vi "梦幻城堡C1~3界面.vi"() -> ()   [LabVIEW 2016, in "环境动力监测库.lvlib" / "UPS库.lvlib"]
uses:
  <vilib>/Utility/config.llb/NI_LVConfig.lvlib
  <vilib>/ptbypt/NI_PtbyPt.lvlib
panel:
  out "关机倒计时":i32
  out "关闭中":bool
  out "通信指示":bool
  out "UPS状态":T1
  in  "关机":bool
  in  "重开串口":bool
  out "Temperature":dbl
  out "Battery voltage":dbl
  out "I/P frequency HZ":dbl
  out "O/P load %":dbl
  out "O/P voltage":dbl
  out "I/P fault voltage":dbl
  out "I/P voltage":dbl
  # "UPS-梦幻城堡C1~3"
  # "输入电压V"
  # "输入故障电压V"
  # "输出电压V"
  # "输出电流A"
  # "输入频率HZ"
  # "电池电压V"
  # "UPS温度℃"
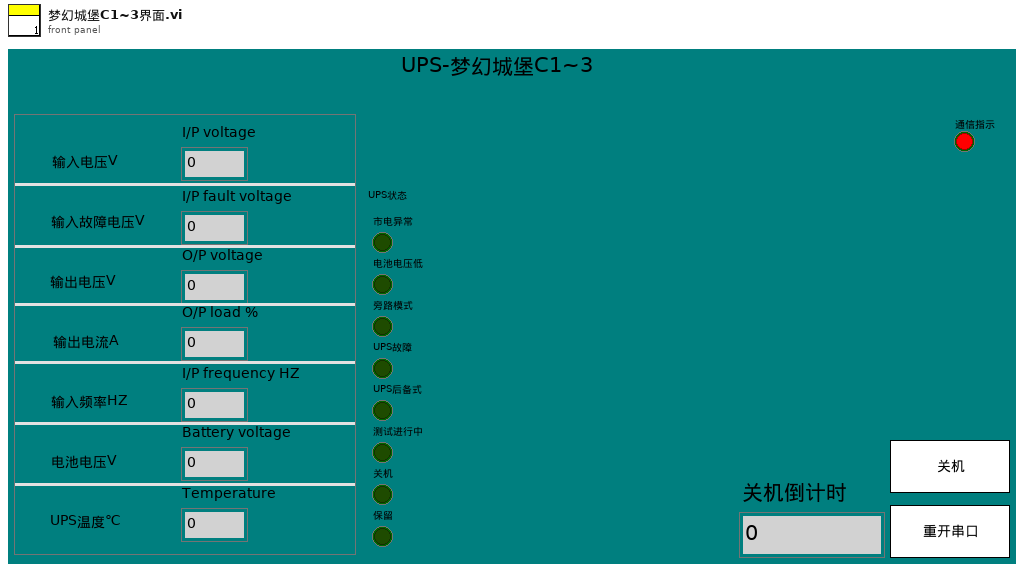
[diagram p1: front panel]
types:
  T1 = cluster{"市电异常":bool, "电池电压低":bool, "旁路模式":bool, "UPS故障":bool, "UPS后备式":bool, "测试进行中":bool, "关机":bool, "保留":bool}
  T2 = cluster{"枚举":enum16{"open", "read", "write", "close"}, "写入缓冲区":string}
  T3 = cluster{"时间标识":timestamp, "设备":string, "日志信息":string}
  T4 = cluster{"I/P voltage":dbl, "I/P fault voltage":dbl, "O/P voltage":dbl, "O/P load %":dbl, "I/P frequency HZ":dbl, "Battery voltage":dbl, "Temperature":dbl, "U":string}
  T5 = cluster{"[0]":bool, "[1]":bool, "[2]":bool, "[3]":bool, "[4]":bool, "[5]":bool, "[6]":bool, "[7]":bool}
  T6 = typedef "NI_LVConfig.lvlib/Config Data RefNum.ctl" = refnum<k1>
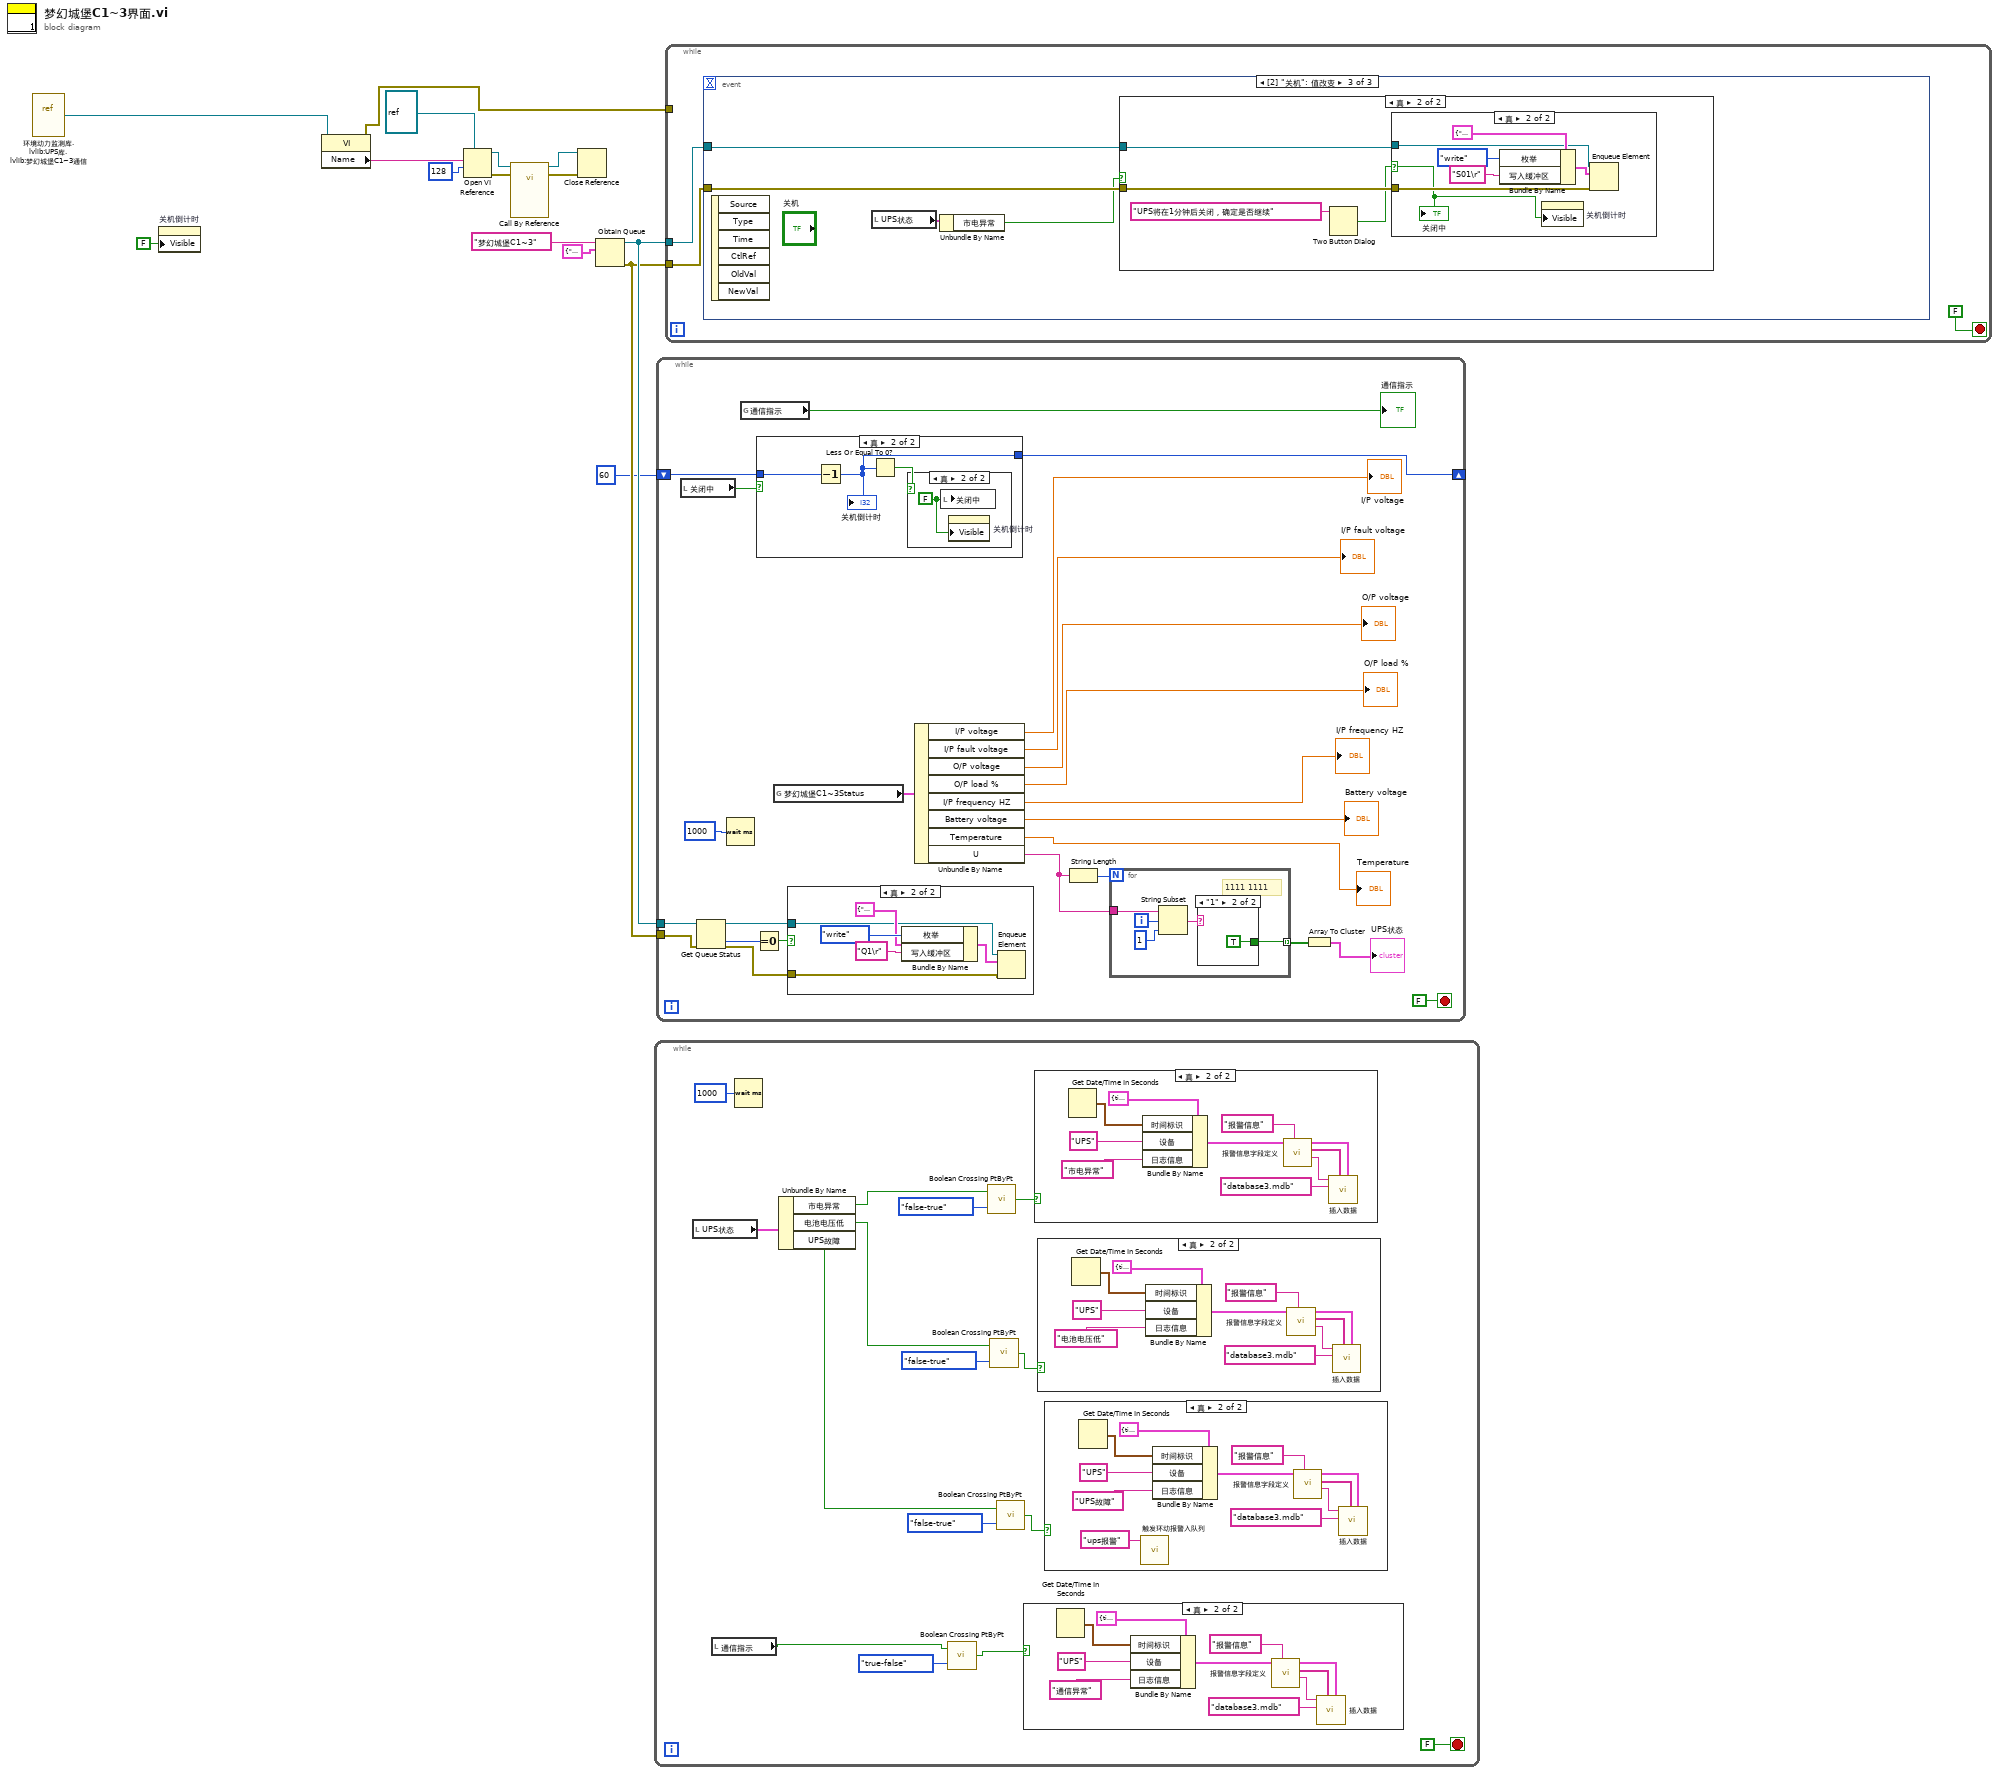
[diagram p0: block diagram]
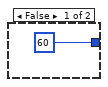
[diagram p7: hidden frame]
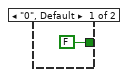
[diagram p9: hidden frame]
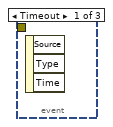
[diagram p10: hidden frame]
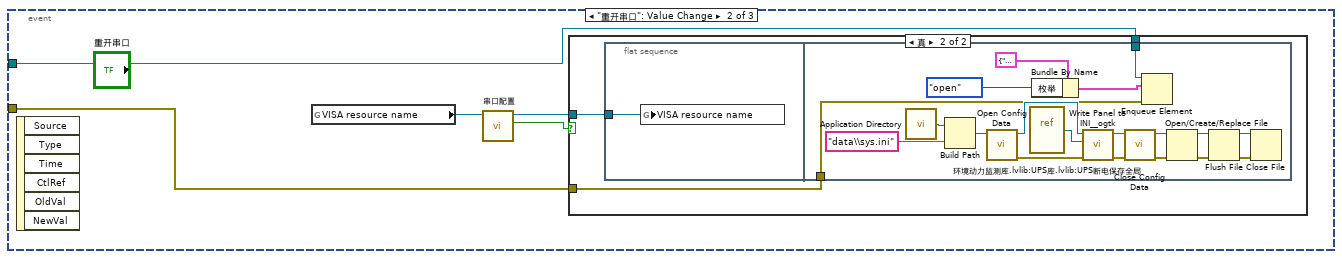
[diagram p11: hidden frame]
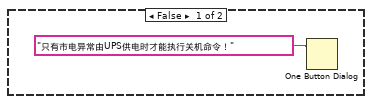
[diagram p13: hidden frame]
diagram:
  n1 = vi-ref "环境动力监测库.lvlib:UPS库.lvlib:梦幻城堡C1~3通信.vi"() -> (w8:refnum<vi>)
  n2 = property on="关机倒计时" class="DigNum (严格)"("Visible"=FALSE ("可见")) -> ()  [unwired: 2 in, 2 out]
  n3 = property class="VI"(reference=w8) -> (error out=w2:errorcluster, "Name"=w9:string)  [unwired: 1 in, 1 out]
  n4 = Open VI Reference(type specifier VI Refnum (for type only)=refnum<vi> refnum, vi path=w9, options=128 ("选项")) -> (vi reference=w11:refnum<vi>, error out=w13:errorcluster)  [unwired: 3 in]
  n5 = call-by-ref "?"(reference=w11, error in=w13) -> (reference out=w15:refnum<vi>, error out=w14:errorcluster)  [unwired: 12 in]
  n6 = Close Reference(reference=w15, error in (no error)=w14) -> ()  [unwired: 1 out]
  n7 = Obtain Queue(name (unnamed)="梦幻城堡C1~3" ("名称（未命名）"), element data type=T2 {"枚举"=enum."open", "写入缓冲区"=""}) -> (queue out=w5:refnum<queue>, error out=w4:errorcluster)  [unwired: 3 in, 1 out]
  n8 = while {
    stop <- FALSE stop-if-true
    n9 = local read "UPS状态"() -> (w28:T1)
    n10 = local read "通信指示"() -> (w16:bool)
    n11 = Wait (ms)(milliseconds to wait=u32 1000 ("等待时间（毫秒）")) -> ()  [unwired: 1 out]
    n12 = Unbundle By Name(w28) -> ("市电异常"=w25:bool, "电池电压低"=w20:bool, "UPS故障"=w19:bool)
    n13 = call <vilib>:"Boolean Crossing PtByPt.vi"("direction"=enum16{"either", "false-true", "true-false"}."true-false", "input"=w16) -> ("crossing"=w17:bool)  [unwired: 1 in]
    n14 = call <vilib>:"Boolean Crossing PtByPt.vi"("direction"=enum16{"either", "false-true", "true-false"}."false-true", "input"=w25) -> ("crossing"=w26:bool)  [unwired: 1 in]
    n15 = call <vilib>:"Boolean Crossing PtByPt.vi"("direction"=enum16{"either", "false-true", "true-false"}."false-true", "input"=w20) -> ("crossing"=w23:bool)  [unwired: 1 in]
    n16 = call <vilib>:"Boolean Crossing PtByPt.vi"("direction"=enum16{"either", "false-true", "true-false"}."false-true", "input"=w19) -> ("crossing"=w22:bool)  [unwired: 1 in]
    n17 = case shown="真" w17 {
      frame False {
      }
      frame True {
        n18 = Get Date/Time In Seconds() -> (seconds since 1Jan1904=w39:timestamp)
        n19 = Bundle By Name(cluster=T3 {"时间标识"=timestamp(0 s since 1904-01-01), "设备"="", "日志信息"=""} ("data in"), "时间标识"=w39, "设备"="UPS", "日志信息"="通信异常") -> (w38:T3)
        n20 = call "报警信息字段定义.vi"("table输入"="报警信息", "data in"=w38) -> ("table输出"=w34:string, "columns"=w33:string[], "data out"=w32:T3)  [unwired: 7 in]
        n21 = call "插入数据.vi"("data"=w32, "columns"=w33, "database"="database3.mdb", "table"=w34) -> ()  [unwired: 7 in, 1 out]
      }
    }
    n22 = case shown="真" w26 {
      frame False {
      }
      frame True {
        n23 = Get Date/Time In Seconds() -> (seconds since 1Jan1904=w70:timestamp)
        n24 = Bundle By Name(cluster=T3 {"时间标识"=timestamp(0 s since 1904-01-01), "设备"="", "日志信息"=""} ("data in"), "时间标识"=w70, "设备"="UPS", "日志信息"="市电异常") -> (w69:T3)
        n25 = call "报警信息字段定义.vi"("table输入"="报警信息", "data in"=w69) -> ("table输出"=w65:string, "columns"=w64:string[], "data out"=w63:T3)  [unwired: 7 in]
        n26 = call "插入数据.vi"("data"=w63, "columns"=w64, "database"="database3.mdb", "table"=w65) -> ()  [unwired: 7 in, 1 out]
      }
    }
    n27 = case shown="真" w23 {
      frame False {
      }
      frame True {
        n28 = Get Date/Time In Seconds() -> (seconds since 1Jan1904=w60:timestamp)
        n29 = Bundle By Name(cluster=T3 {"时间标识"=timestamp(0 s since 1904-01-01), "设备"="", "日志信息"=""} ("data in"), "时间标识"=w60, "设备"="UPS", "日志信息"="电池电压低") -> (w59:T3)
        n30 = call "报警信息字段定义.vi"("table输入"="报警信息", "data in"=w59) -> ("table输出"=w55:string, "columns"=w54:string[], "data out"=w53:T3)  [unwired: 7 in]
        n31 = call "插入数据.vi"("data"=w53, "columns"=w54, "database"="database3.mdb", "table"=w55) -> ()  [unwired: 7 in, 1 out]
      }
    }
    n32 = case shown="真" w22 {
      frame False {
      }
      frame True {
        n33 = Get Date/Time In Seconds() -> (seconds since 1Jan1904=w50:timestamp)
        n34 = call "触发环动报警入队列.vi"("报警内容"="ups报警") -> ()  [unwired: 11 in]
        n35 = Bundle By Name(cluster=T3 {"时间标识"=timestamp(0 s since 1904-01-01), "设备"="", "日志信息"=""} ("data in"), "时间标识"=w50, "设备"="UPS", "日志信息"="UPS故障") -> (w49:T3)
        n36 = call "报警信息字段定义.vi"("table输入"="报警信息", "data in"=w49) -> ("table输出"=w45:string, "columns"=w44:string[], "data out"=w43:T3)  [unwired: 7 in]
        n37 = call "插入数据.vi"("data"=w43, "columns"=w44, "database"="database3.mdb", "table"=w45) -> ()  [unwired: 7 in, 1 out]
      }
    }
  }
  n38 = while {
    tunnel: w5 -> [w76]
    tunnel: w4 -> [w75]
    shift-right: [w78] -> _
    shift-left: 60 -> [w79]
    stop <- FALSE stop-if-true
    n39 = local read "关闭中"() -> (w80:bool)
    n40 = Get Queue Status(queue=w76, error in (no error)=w75) -> (queue out=w74:refnum<queue>, error out=w73:errorcluster, # elements in queue=w77:i32)  [unwired: 1 in, 5 out]
    n41 = Wait (ms)(milliseconds to wait=u32 1000 ("等待时间（毫秒）")) -> ()  [unwired: 1 out]
    n42 = global read "UPS内部交互全局.vi" "通信指示"() -> (→"通信指示":bool)
    n43 = Equal To 0?(x=w77) -> (x = 0?=w72:bool)
    n44 = case shown="真" w80 {
      tunnel: w79 -> [_ w105]
      tunnel: [60 w104] -> w78
      frame False {
      }
      frame True {
        n45 = Decrement(x=w105) -> (x-1=w104:i32)
        "关机倒计时" <- w104
        n46 = Less Or Equal To 0?(x=w104) -> (x <= 0?=w103:bool)
        n47 = case shown="真" w103 {
          frame False {
          }
          frame True {
            w106 = FALSE ("关闭中")
            n48 = local write "关闭中"(w106) -> ()
            n49 = property on="关机倒计时" class="DigNum (严格)"("Visible"=w106) -> ()  [unwired: 2 in, 2 out]
          }
        }
      }
    }
    n50 = global read "UPS内部交互全局.vi" "梦幻城堡C1~3Status"() -> (w93:T4)
    n51 = case shown="真" w72 {
      tunnel: w74 -> [_ w97]
      tunnel: w73 -> [_ w96]
      frame False {
      }
      frame True {
        n52 = Bundle By Name(cluster=T2 {"枚举"=enum."open", "写入缓冲区"=""}, "枚举"=enum16{"open", "read", "write", "close"}."write", "写入缓冲区"="Q1\r") -> (w100:T2)
        n53 = Enqueue Element(queue=w97, element=w100, error in (no error)=w96) -> ()  [unwired: 1 in, 3 out]
      }
    }
    n54 = Unbundle By Name(w93) -> ("I/P voltage"=→"I/P voltage":dbl, "I/P fault voltage"=→"I/P fault voltage":dbl, "O/P voltage"=→"O/P voltage":dbl, "O/P load %"=→"O/P load %":dbl, "I/P frequency HZ"=→"I/P frequency HZ":dbl, "Battery voltage"=→"Battery voltage":dbl, "Temperature"=→"Temperature":dbl, "U"=w81:string)
    n55 = String Length(string=w81) -> (length=w83:i32)
    n56 = for {
      N: w83 -> [_]
      tunnel: w81 -> [w111]
      tunnel: [w107] -> w82 mode=indexing
      i -> [w109]
      # "1111 1111"
      n57 = String Subset(string=w111, offset (0)=w109, length (rest)=1 ("长度（剩余）")) -> (substring=w108:string)
      n58 = case shown="\"1\"" w108 {
        tunnel: [FALSE TRUE] -> w107
        frame "0", Default {
        }
        frame "1" {
        }
      }
    }
    n59 = Array To Cluster(array=w82) -> (cluster=→"UPS状态":T5)
  }
  n60 = while {
    tunnel: w4 -> [w115]
    tunnel: w5 -> [w114]
    tunnel: w2 -> [_]
    stop <- FALSE stop-if-true
    n61 = event shown="[2] \"关机\": 值改变" {
      selector: _ -> [_ _ _]
      dyn-events: _ -> [_ _ _]
      timeout: _ -> [_ _ _]
      tunnel: w115 -> [_ w117 w147]
      tunnel: w114 -> [_ w118 w148]
      event Timeout {
        n62 = event-data() -> ()  [unwired: 1 in, 3 out]
      }
      event "重开串口": Value Change {
        n63 = event-data() -> ()  [unwired: 1 in, 6 out]
        n64 = global read "UPS断电保存全局.vi" "VISA resource name"() -> (w121:refnum<visa-resource-name>)
        n65 = call "串口配置.vi"("请选择串口:"=w121) -> ("确认 2"=w120:bool, "请选择串口: 2"=w119:refnum<visa-resource-name>)  [unwired: 9 in]
        n66 = case shown="真" w120 {
          tunnel: w119 -> [_ w124]
          tunnel: w118 -> [_ w123]
          tunnel: w117 -> [_ w122]
          frame False {
          }
          frame True {
            n67 = flat-sequence {
              tunnel: w124 -> [w125]
              tunnel: w123 -> [w127]
              tunnel: w122 -> [w126]
              frame #0 {
                n68 = global write "UPS断电保存全局.vi" "VISA resource name"(w125) -> ()
              }
              frame #1 {
                n69 = call <vilib>:"Application Directory.vi"() -> ("Application Directory"=w132:path)
                n70 = Build Path(base path=w132, name or relative path="data\\sys.ini" ("名称或相对路径")) -> (appended path=w133:path)
                n71 = call <vilib>:"Open Config Data.vi"("configuration file path"=w133) -> ("error out"=w137:errorcluster, "refnum"=w134:T6)  [unwired: 8 in, 1 out]
                n72 = vi-ref "环境动力监测库.lvlib:UPS库.lvlib:UPS断电保存全局.vi"() -> (w135:refnum<vi>)
                n73 = Bundle By Name(cluster=T2 {"枚举"=enum."open", "写入缓冲区"=""}, "枚举"=enum16{"open", "read", "write", "close"}."open") -> (w130:T2)
                n74 = call <userlib>:"Write Panel to INI__ogtk.vi"("error in (no error)"=w137, "VI ref"=w135, "refnum"=w134) -> ("error out"=w138:errorcluster, "refnum out"=w136:T6)  [unwired: 7 in]
                n75 = call <vilib>:"Close Config Data.vi"("error in (no error)"=w138, "refnum"=w136) -> ("error out"=w143:errorcluster, "file path"=w144:path)  [unwired: 8 in]
                n76 = Enqueue Element(queue=w127, element=w130, error in (no error)=w126) -> ()  [unwired: 1 in, 3 out]
                n77 = Open/Create/Replace File(file path (use dialog)=w144, error in=w143) -> (refnum out=w140:refnum<file>, error out=w139:errorcluster)  [unwired: 4 in, 1 out]
                n78 = Flush File(refnum=w140, error in=w139) -> (refnum out=w141:refnum<file>, error out=w142:errorcluster)
                n79 = Close File(refnum=w141, error in=w142) -> ()  [unwired: 2 out]
              }
            }
          }
        }
      }
      event "关机": Value Change {
        n80 = event-data() -> ()  [unwired: 1 in, 6 out]
        n81 = local read "UPS状态"() -> (w146:T1)
        n82 = Unbundle By Name(w146) -> ("市电异常"=w145:bool)
        n83 = case shown="真" w145 {
          tunnel: w148 -> [_ w153]
          tunnel: w147 -> [_ w152]
          frame False {
            n84 = One Button Dialog(message="只有市电异常由UPS供电时才能执行关机命令！" ("消息")) -> ()  [unwired: 1 in, 1 out]
          }
          frame True {
            n85 = Two Button Dialog(message="UPS将在1分钟后关闭，确定是否继续" ("消息")) -> (T button?=w150:bool)  [unwired: 2 in]
            n86 = case shown="真" w150 {
              selector: w150 -> [_ w154]
              tunnel: w153 -> [_ w157]
              tunnel: w152 -> [_ w156]
              frame False {
              }
              frame True {
                n87 = Bundle By Name(cluster=T2 {"枚举"=enum."open", "写入缓冲区"=""}, "枚举"=enum16{"open", "read", "write", "close"}."write", "写入缓冲区"="S01\r") -> (w158:T2)
                n88 = property on="关机倒计时" class="DigNum (严格)"("Visible"=w154) -> ()  [unwired: 2 in, 2 out]
                n89 = Enqueue Element(queue=w157, element=w158, error in (no error)=w156) -> ()  [unwired: 1 in, 3 out]
                "关闭中" <- w154
              }
            }
          }
        }
      }
    }
  }
